vi "DAQmx Write (Counter Frequency 1Chan 1Samp).vi"(0 "task/channels in":refnum<k21>, 1 "auto start":bool=TRUE, 5 "frequency":dbl=1.0 format="%_6g", 7 "duty cycle":dbl=0.5 format="%_6g", 9 "timeout":dbl=10.0 format="%0.2f", 11 "error in":errorcluster) -> (4 "task out":refnum<k21>, 10 "number of samples written per channel":u32, 15 "error out":errorcluster)   [LabVIEW 2024]
doc: "Writes a new pulse frequency and duty cycle to a counter output task that contains a single channel."
uses:
  nilvaiu.dll
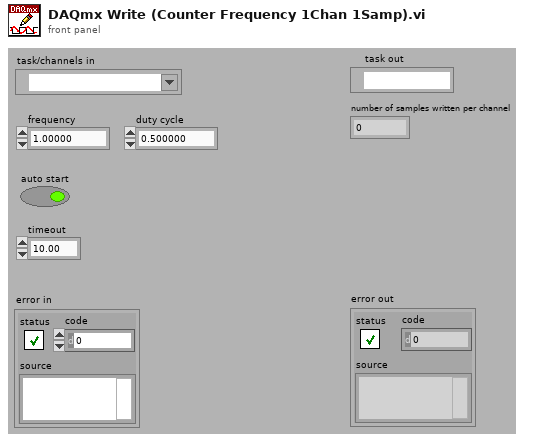
[diagram p1: front panel]
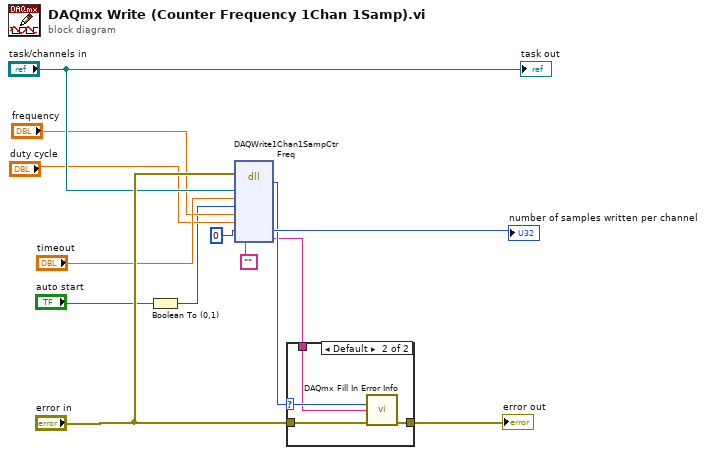
[diagram p0: block diagram]
diagram:
  n1 = Boolean To (0,1)(Boolean="auto start") -> (0, 1=w4:i16)
  n2 = dll-call lib="nilvaiu.*" fn="DAQWrite1Chan1SampCtrFreq"(error in="error in", "taskID"="task/channels in", "timeout"="timeout", "autoStart"=w4, "frequency"="frequency", "dutyCycle"="duty cycle", "numSamplesWriten"=u32 0, "extendedErrorInfo"="") -> (w5:i32, "numSamplesWriten"=→"number of samples written per channel":u32, "extendedErrorInfo"=w1:string)  [unwired: 5 in, 4 out]
  n3 = case shown="Default" w5 {
    selector: w5 -> [_ w16]
    tunnel: "error in" -> [w14 w18]
    tunnel: [w14 w17] -> w11
    tunnel: w1 -> [_ w15]
    frame 0 {
    }
    frame Default {
      n4 = call "DAQmx Fill In Error Info.vi"("status code"=w16, "extended error info"=w15, "error in"=w18) -> ("error out"=w17:errorcluster)  [unwired: 1 in, 11 out]
    }
  }
  "error out" <- w11
  "task out" <- "task/channels in"
